vi "fgv_9467_Config.vi"(7 "cmd":T1=enum."write", 11 "cDAQ-9467 Config":tag="cDAQ9185-213AA55Mod1/port0") -> (3 "cDAQ-9467 Config 2":tag="cDAQ9185-213AA55Mod1/port0")   [LabVIEW 2019]
uses:
  _ctrl/rw.ctl
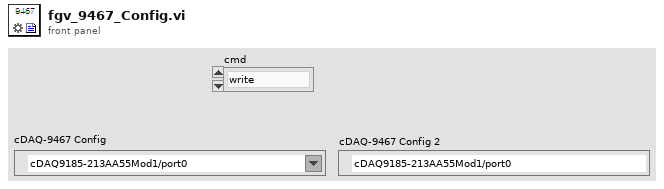
[diagram p1: front panel]
types:
  T1 = typedef "rw.ctl" = enum16{"read", "write"}
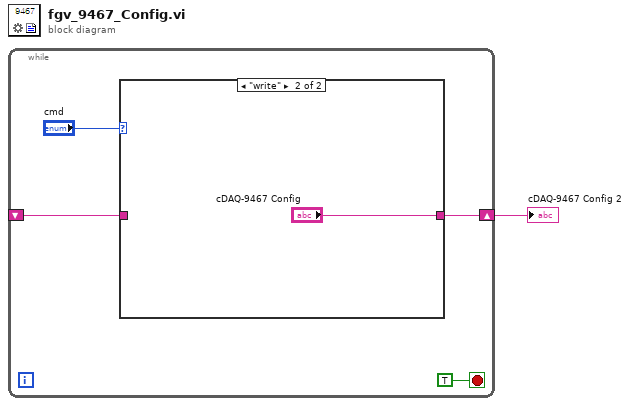
[diagram p0: block diagram]
diagram:
  n1 = while {
    shift-right: [w3] -> w1
    shift-left: _ -> [w2]
    stop <- TRUE stop-if-true
    n2 = case shown="\"write\"" "cmd" {
      tunnel: [w6 "cDAQ-9467 Config"] -> w3
      tunnel: w2 -> [w6 _]
      frame "read", Default {
      }
      frame "write" {
      }
    }
  }
  "cDAQ-9467 Config 2" <- w1
